vi "SDSU_MemRead.vi"(5 "type":string, 7 "board dest":i16, 8 "error in (no error)":errorcluster, 10 "memin":string, 11 "fd":i32) -> (0 "error out":errorcluster, 2 "values":string, 3 "fd out":i32)   [LabVIEW 2016]
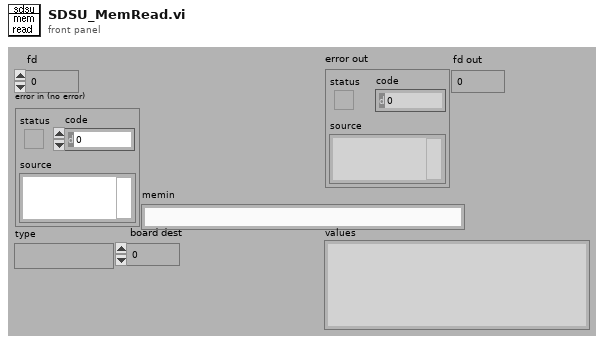
[diagram p1: front panel]
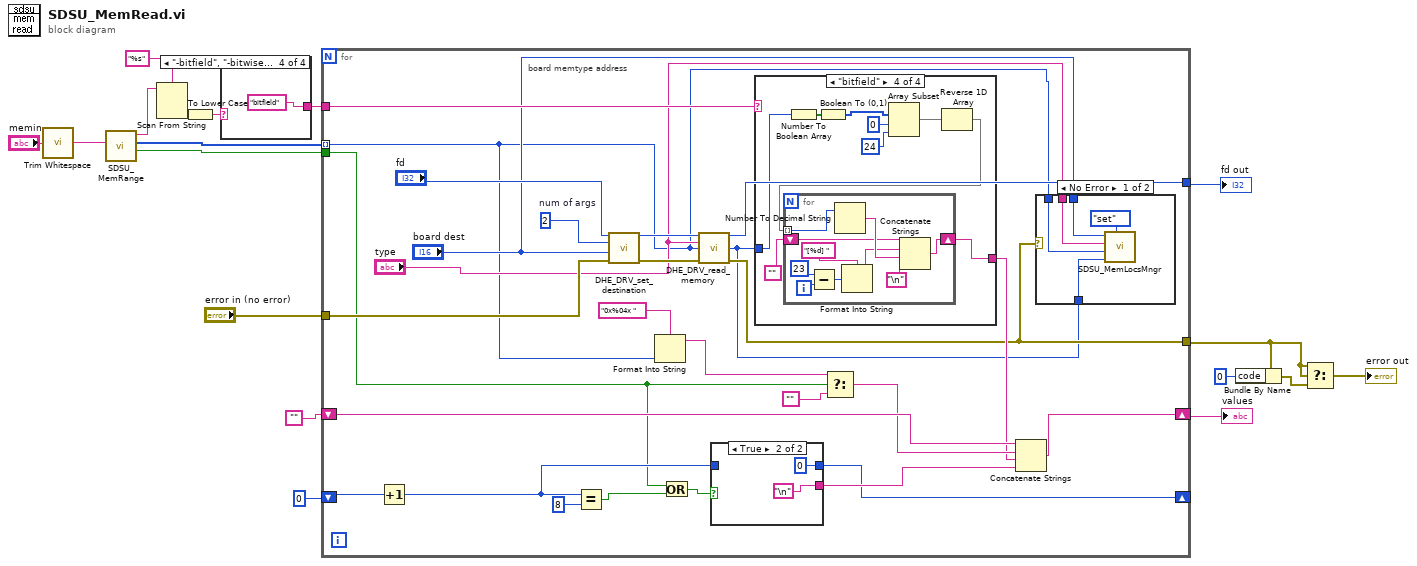
[diagram p0: block diagram]
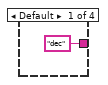
[diagram p2: hidden frame]
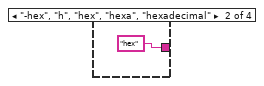
[diagram p3: hidden frame]
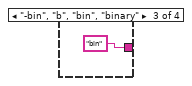
[diagram p4: hidden frame]
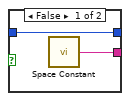
[diagram p6: hidden frame]
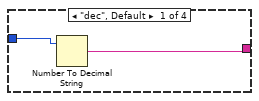
[diagram p7: hidden frame]
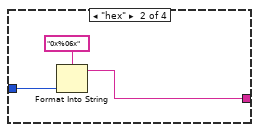
[diagram p8: hidden frame]
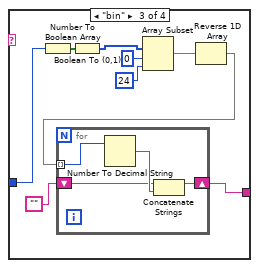
[diagram p9: hidden frame]
diagram:
  n1 = call <vilib>:"Trim Whitespace.vi"("string"="memin") -> ("trimmed string"=w2:string)  [unwired: 1 in]
  n2 = call "SDSU_MemRange.vi"("memin"=w2) -> ("inc adds"=w15:bool, "address"=w16:i32[], "remaining string"=w14:string)  [unwired: 8 out]
  n3 = Scan From String(format string="%s", input string=w14) -> (output 1=w12:string)  [unwired: 2 in, 4 out]
  n4 = To Lower Case(string=w12) -> (all lower case string=w11:string)
  n5 = case shown="\"-bitfield\", \"-bitwise\", \"bitfield\", \"bitwise\", \"byfield\", \"field\"" w11 {
    tunnel: ["dec" "hex" "bin" "bitfield"] -> w1
    frame Default {
    }
    frame "-hex", "h", "hex", "hexa", "hexadecimal" {
    }
    frame "-bin", "b", "bin", "binary" {
    }
    frame "-bitfield", "-bitwise", "bitfield", "bitwise", "byfield", "field" {
    }
  }
  n6 = for {
    tunnel: [w47] -> w18
    tunnel: w16 -> [w24] mode=indexing
    tunnel: w15 -> [w29]
    shift-right: [w37] -> w7
    shift-left: "" -> [w40]
    tunnel: "error in (no error)" -> [w43]
    shift-right: [w31] -> _
    shift-left: 0 -> [w36]
    tunnel: [w27] -> w5
    tunnel: w1 -> [w28]
    w46 = 2  # num of args
    # "board memtype address"
    n7 = Increment(x=w36) -> (x+1=w33:i32)
    n8 = Equal?(x=w33, y=8) -> (x = y?=w34:bool)
    n9 = call "DHE_DRV_set_destination.vi"("fd"="fd", "num of args"=w46, "board dest"="board dest", "error in (no error)"=w43) -> ("fd out"=w48:i32, "error out"=w49:errorcluster)  [unwired: 10 out]
    n10 = Format Into String(format string="0x%04x ", w24) -> (resulting string=w42:string)  [unwired: 2 in, 1 out]
    n11 = Or(x=w29, y=w34) -> (x .or. y?=w30:bool)
    n12 = call "DHE_DRV_read_memory.vi"("fd"=w48, "type"="type", "address"=w24, "error in (no error)"=w49) -> ("fd"=w47:i32, "return value"=w23:i32, "error out"=w27:errorcluster)  [unwired: 9 out]
    n13 = case shown="True" w30 {
      tunnel: w33 -> [w55 _]
      tunnel: [w56 "\n"] -> w32
      tunnel: [w55 0] -> w31
      frame False {
        n14 = call <vilib>:"Space Constant.vi"() -> ("String"=w56:string)
      }
      frame True {
      }
    }
    n15 = case shown="\"bitfield\"" w28 {
      tunnel: w23 -> [w60 w63 w72 w85]
      tunnel: [w59 w61 w64 w78] -> w38
      frame "dec", Default {
        n16 = Number To Decimal String(number=w60) -> (decimal integer string=w59:string)  [unwired: 1 out]
      }
      frame "hex" {
        n17 = Format Into String(format string="0x%06x", w63) -> (resulting string=w61:string)  [unwired: 2 in, 1 out]
      }
      frame "bin" {
        n18 = Number To Boolean Array(number=w72) -> (Boolean array=w71:bool[])
        n19 = Boolean To (0,1)(Boolean=w71) -> (0, 1=w67:i16[])
        n20 = Array Subset(array=w67, index=0, length=24) -> (w66:i16[])
        n21 = Reverse 1D Array(array=w66) -> (reversed array=w65:i16[])
        n22 = for {
          tunnel: w65 -> [w76] mode=indexing
          shift-right: [w73] -> w64
          shift-left: "" -> [w74]
          n23 = Number To Decimal String(number=w76) -> (decimal integer string=w75:string)  [unwired: 1 out]
          n24 = Concatenate Strings(w74, w75) -> (w73:string)
        }
      }
      frame "bitfield" {
        n25 = Number To Boolean Array(number=w85) -> (Boolean array=w84:bool[])
        n26 = Boolean To (0,1)(Boolean=w84) -> (0, 1=w81:i16[])
        n27 = Array Subset(array=w81, index=0, length=24) -> (w80:i16[])
        n28 = Reverse 1D Array(array=w80) -> (reversed array=w79:i16[])
        n29 = for {
          tunnel: w79 -> [w95] mode=indexing
          shift-right: [w90] -> w78
          shift-left: "" -> [w89]
          i -> [w87]
          n30 = Subtract(x=23, y=w87) -> (x-y=w86:i32)
          n31 = Number To Decimal String(number=w95) -> (decimal integer string=w94:string)  [unwired: 1 out]
          n32 = Format Into String(format string="[%d] ", w86) -> (resulting string=w91:string)  [unwired: 2 in, 1 out]
          n33 = Concatenate Strings(w89, w91, w94, "\n") -> (w90:string)
        }
      }
    }
    n34 = Select(t=w42, s=w29, f="") -> (s? t:f=w39:string)
    n35 = Concatenate Strings(w40, w39, w38, w32) -> (w37:string)
    n36 = case shown="No Error" w27 {
      tunnel: "board dest" -> [w53 _]
      tunnel: "type" -> [w52 _]
      tunnel: w24 -> [w51 _]
      tunnel: w23 -> [w50 _]
      frame No Error {
        n37 = call "SDSU_MemLocsMngr.vi"("action"=enum16{"set", "get", "clear"}."set", "value"=w50, "address"=w51, "type"=w52, "board"=w53) -> ()  [unwired: 5 in, 2 out]
      }
      frame Error {
      }
    }
  }
  "fd out" <- w18
  "values" <- w7
  n38 = Bundle By Name(cluster=w5, "code"=0) -> (w4:errorcluster)
  n39 = Select(t=w5, s=w5, f=w4) -> (s? t:f=→"error out":errorcluster)
